vi "Hold Robot.vi"(11 "Reset Encoders?":bool) -> (3 "Speed Output":cluster{"output":dbl, "output":dbl})   [LabVIEW 2013]
uses:
  <vilib>/addons/control/pid/pid.llb/PID (DBL).vi
  <vilib>/addons/control/pid/NI_PID_pid.lvlib
panel:
  in  "PID gains":T1={"proportional gain (Kc)"=1.0, "integral time (Ti, min)"=0.01, "derivative time (Td, min)"=0.0} {"derivative time (Td, min)" format="%.3f"; "integral time (Ti, min)" format="%.3f"; "proportional gain (Kc)" format="%.3f"}
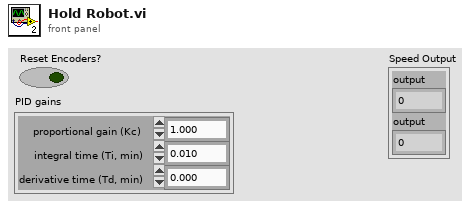
[diagram p1: front panel]
types:
  T1 = cluster{"proportional gain (Kc)":dbl, "integral time (Ti, min)":dbl, "derivative time (Td, min)":dbl}
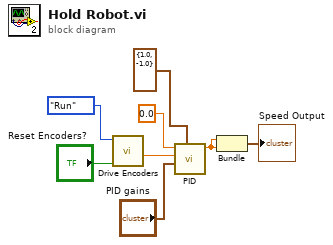
[diagram p0: block diagram]
diagram:
  n1 = call "Drive Encoders.vi"("Reset Encoders?"="Reset Encoders?", "Mode"=enum16{"Init", "Run", "End"}."Run") -> ("Average Distance"=w5:dbl)  [unwired: 4 in, 5 out]
  n2 = call-poly <vilib>:"PID.vi"("output range"=cluster{"output high":dbl, "output low":dbl} {"output high"=1.0, "output low"=-1.0}, "PID gains"="PID gains", "process variable"=w5, "setpoint"=0.0) -> ("output"=w2:dbl)  [unwired: 6 in, 1 out]
  n3 = Bundle("output"=w2, "output"=w2) -> (→"Speed Output":cluster{"output":dbl, "output":dbl})  [unwired: 1 in]
